vi "motor.vi"() -> ()   [LabVIEW 2016]
uses:
  <vilib>/myRIO/Common/Instrument Driver Framework/myRIO v1.0/Encoder/typedefs/Encoder Signal Mode.ctl
  <vilib>/myRIO/Instrument Drivers/Onboard IO/DIO/typedefs/DIO Reference.ctl
  <vilib>/myRIO/Common/Instrument Driver Framework/Utilities/typedefs/myRIO Generic Hardware Reference.ctl
  <vilib>/myRIO/Common/Instrument Driver Framework/Utilities/typedefs/Hardware Version Enum.ctl
  <vilib>/myRIO/Common/Instrument Driver Framework/Utilities/typedefs/myRIO v1.0 Reference.ctl
  <vilib>/myRIO/Common/Instrument Driver Framework/Utilities/typedefs/Generic FPGA Reference.ctl
  <vilib>/myRIO/Common/Instrument Driver Framework/myRIO v1.0/DIO/typedefs/DIO Channels List.ctl
  <vilib>/myRIO/Common/Instrument Driver Framework/myRIO v1.0/DIO/typedefs/DIO Channels Enum.ctl
  <vilib>/userdefined/High Color/nirio_resource_hc.ctl
  <vilib>/myRIO/Instrument Drivers/Onboard IO/PWM/typedefs/PWM Reference.ctl
  <vilib>/myRIO/Common/Instrument Driver Framework/myRIO v1.0/PWM/typedefs/PWM Channels Enum.ctl
  <vilib>/myRIO/Instrument Drivers/Onboard IO/PWM/typedefs/PWM Configuration.ctl
  <vilib>/myRIO/Common/Instrument Driver Framework/myRIO v1.0/Encoder/typedefs/Encoder Configuration v1.0.ctl
  <vilib>/myRIO/Instrument Drivers/Onboard IO/Encoder/typedefs/Encoder Reference.ctl
  <vilib>/myRIO/Common/Instrument Driver Framework/myRIO v1.0/Encoder/typedefs/Encoder Channels Enum.ctl
  <vilib>/myRIO/Common/Instrument Driver Framework/Utilities/vis/Is FPGA Ref Available.vi
  <vilib>/myRIO/Common/Instrument Driver Framework/myRIO v1.0/DIO/vis/myRIO v1.1 Open DIO.vi
  <vilib>/myRIO/Instrument Drivers/Onboard IO/DIO/vis/Write.vi
  <vilib>/myRIO/Common/Instrument Driver Framework/myRIO v1.0/PWM/vis/myRIO v1.1 Open PWM.vi
  <vilib>/myRIO/Common/Instrument Driver Framework/myRIO v1.0/Encoder/vis/myRIO v1.1 Open Encoder.vi
  <vilib>/myRIO/Common/Instrument Driver Framework/Utilities/vis/Validate Channels.vi
  <vilib>/myRIO/Common/Instrument Driver Framework/myRIO v1.0/DIO/vis/myRIO v1.0 Reserve DIO.vi
  <vilib>/myRIO/Common/Instrument Driver Framework/myRIO v1.0/PWM/vis/myRIO v1.0 Reserve PWM.vi
  <vilib>/myRIO/Common/Instrument Driver Framework/myRIO v1.0/Encoder/vis/myRIO v1.0 Reserve Encoder.vi
  <vilib>/myRIO/Common/Instrument Driver Framework/myRIO v1.0/Encoder/vis/myRIO v1.0 Close Encoder.vi
  <vilib>/myRIO/Common/Instrument Driver Framework/myRIO v1.0/PWM/vis/myRIO v1.0 Close PWM.vi
  <vilib>/myRIO/Common/Instrument Driver Framework/myRIO v1.0/Resource Manager/vis/myRIO v1.0 Reserve Channel List.vi
  <vilib>/myRIO/Common/Instrument Driver Framework/myRIO v1.0/DIO/vis/myRIO v1.0 Build MUX Configuration DIO.vi
  <vilib>/myRIO/Common/Instrument Driver Framework/myRIO v1.0/PWM/vis/myRIO v1.0 Build MUX Configuration PWM.vi
  <vilib>/myRIO/Common/Instrument Driver Framework/myRIO v1.0/Encoder/vis/myRIO v1.0 Build MUX Configuration Encoder.vi
  <vilib>/myRIO/Common/Instrument Driver Framework/myRIO v1.0/Encoder/vis/myRIO v1.0 Unreserve Encoder.vi
  <vilib>/myRIO/Common/Instrument Driver Framework/myRIO v1.0/PWM/vis/myRIO v1.0 Unreserve PWM.vi
  <vilib>/myRIO/Common/Instrument Driver Framework/myRIO v1.0/Resource Manager/vis/myRIO v1.0 Reserve Channel.vi
  <vilib>/myRIO/Common/Instrument Driver Framework/myRIO v1.0/Resource Manager/vis/myRIO v1.0 Unreserve Channel.vi
  <vilib>/myRIO/Common/Instrument Driver Framework/myRIO v1.0/Resource Manager/vis/myRIO v1.0 Create Configuration List.vi
  <vilib>/myRIO/Common/Instrument Driver Framework/myRIO v1.0/Resource Manager/vis/myRIO v1.0 Unreserve Channel List.vi
  <vilib>/myRIO/Common/Instrument Driver Framework/myRIO v1.0/Resource Manager/vis/myRIO v1.0 Build Mutex Name.vi
  <vilib>/Utility/VariantDataType/GetNumericInfo.vi
  <vilib>/Utility/error.llb/Error Cluster From Error Code.vi
  <vilib>/myRIO/Common/Instrument Driver Framework/myRIO v1.0/myRIO v1.1 Open.vi
  <vilib>/myRIO/Common/Instrument Driver Framework/Utilities/vis/IO Manager.vi
  <vilib>/myRIO/Common/Instrument Driver Framework/Utilities/vis/Configuration Manager.vi
  <vilib>/myRIO/Common/Instrument Driver Framework/myRIO v1.0/Resource Manager/vis/myRIO v1.0 Configure IO.vi
  <vilib>/myRIO/Common/Instrument Driver Framework/myRIO v1.0/myRIO v1.0 Close.vi
  <vilib>/myRIO/Common/Instrument Driver Framework/myRIO v1.0/DIO/vis/myRIO v1.0 Write DIO.vi
  <vilib>/myRIO/Common/Instrument Driver Framework/myRIO v1.0/Encoder/vis/myRIO v1.0 Configure Encoder.vi
  <vilib>/myRIO/Common/Instrument Driver Framework/myRIO v1.0/Encoder/vis/myRIO v1.0 Read Encoder.vi
  <vilib>/addons/control/pid/pid.llb/PID (DBL).vi
  <vilib>/myRIO/Common/Instrument Driver Framework/myRIO v1.0/PWM/vis/myRIO v1.0 Write PWM.vi
  <vilib>/myRIO/Common/Instrument Driver Framework/myRIO v1.0/Encoder/vis/myRIO v1.0 Shutdown Encoder.vi
  <vilib>/myRIO/Common/Instrument Driver Framework/myRIO v1.0/PWM/vis/myRIO v1.0 Shutdown PWM.vi
  <vilib>/myRIO/Express VI/Onboard IO/DO/DO Express VI.xnode
  <vilib>/myRIO/Instrument Drivers/Onboard IO/DIO/vis/myRIO DIO Open.xnode
  <vilib>/myRIO/Instrument Drivers/Onboard IO/Encoder/vis/myRIO Encoder Open.xnode
  <vilib>/myRIO/Instrument Drivers/Onboard IO/PWM/vis/myRIO PWM Open.xnode
  <vilib>/myRIO/Instrument Drivers/Onboard IO/Encoder/Encoder.lvlib
  <vilib>/myRIO/Instrument Drivers/Onboard IO/PWM/PWM.lvlib
  <vilib>/myRIO/Instrument Drivers/Onboard IO/DIO/DIO.lvlib
  <vilib>/addons/control/pid/NI_PID_pid.lvlib
panel:
  out "element":dbl
  in  "Numeric":dbl
  in  "PID gains":T1={"proportional gain (Kc)"=1.0, "integral time (Ti, min)"=0.01, "derivative time (Td, min)"=0.0} {"derivative time (Td, min)" format="%.6f"; "integral time (Ti, min)" format="%.6f"; "proportional gain (Kc)" format="%.4f"}
  out "Waveform Chart":dbl(graph)
  in  "Boolean 2":bool
  out "error out 4":errorcluster
  in  "error in (no error) 4":errorcluster
  in  "Boolean":bool
  out "error out 3":errorcluster
  in  "error in (no error) 3":errorcluster
  out "error out 2":errorcluster
  in  "error in (no error)":errorcluster
  out "Counter Value":i32
  in  "stop":bool
  out "error out":errorcluster
  in  "error in (no error) 2":errorcluster
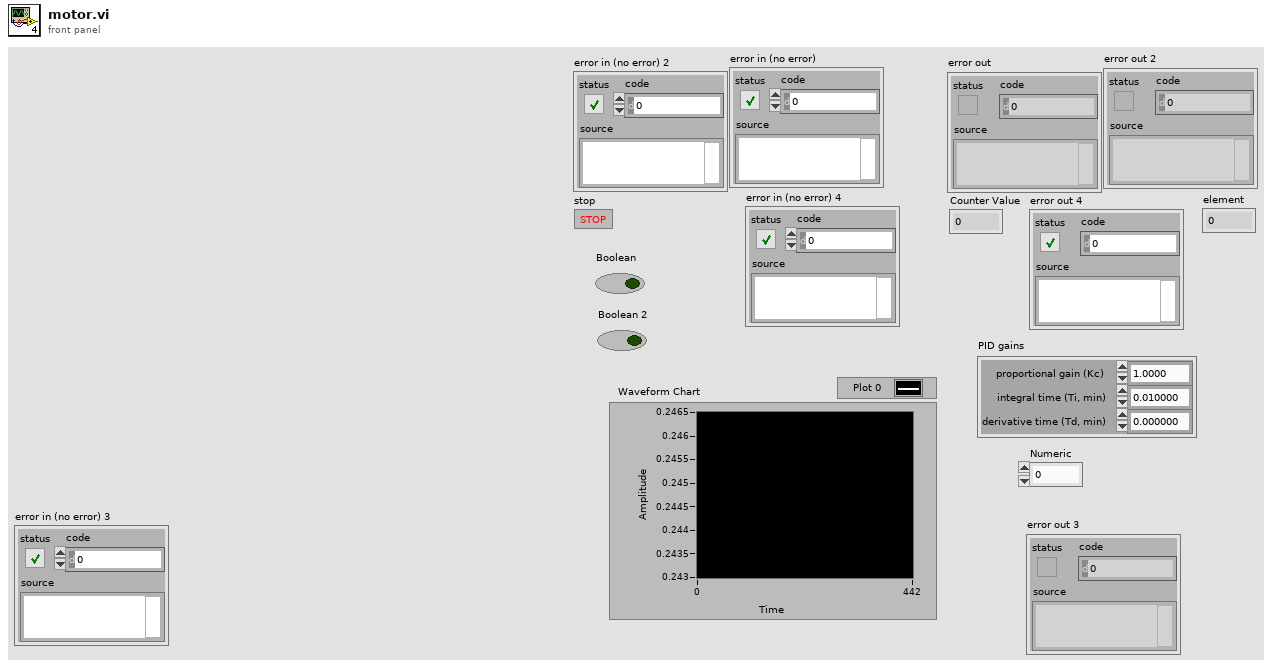
[diagram p1: front panel]
types:
  T1 = cluster{"proportional gain (Kc)":dbl, "integral time (Ti, min)":dbl, "derivative time (Td, min)":dbl}
  T2 = typedef "Encoder Signal Mode.ctl" = enum16{"Quadrature phase signal", "Step and direction signal"}
  T3 = typedef "DIO.lvlib/DIO Reference.ctl" = cluster{"myRIO Reference":T4, "DIO Channels List":T8}
  T4 = typedef "myRIO Generic Hardware Reference.ctl" = cluster{"myRIO Model":T5, "myRIO Hardware Reference":T6}
  T5 = typedef "Hardware Version Enum.ctl" = enum16{"Unknown", "myRIO-1900", "myRIO-1950", "roboRIO", "NI ELVIS RIO CM"}
  T6 = typedef "myRIO v1.0 Reference.ctl" = cluster{"Generic FPGA Reference":T7, "Allow multiple opens":bool}
  T7 = typedef "Generic FPGA Reference.ctl" = refnum<k20>
  T8 = typedef "DIO Channels List.ctl" = T9[]
  T9 = typedef "DIO Channels Enum.ctl" = enum16{"Not Connected", "C/DIO0", "C/DIO1", "C/DIO2", "C/DIO3", "C/DIO4", "C/DIO5", "C/DIO6", "C/DIO7", "A/DIO0", "A/DIO1", "A/DIO2", "A/DIO3", "A/DIO4", "A/DIO5", "A/DIO6", "A/DIO7", "A/DIO8", "A/DIO9", "A/DIO10", "A/DIO11", "A/DIO12", "A/DIO13", "A/DIO14", "A/DIO15", "B/DIO0", "B/DIO1", "B/DIO2", "B/DIO3", "B/DIO4", "B/DIO5", "B/DIO6", "B/DIO7", "B/DIO8", "B/DIO9", "B/DIO10", "B/DIO11", "B/DIO12", "B/DIO13", "B/DIO14", "B/DIO15", "LED0", "LED1", "LED2", "LED3", "Button0", "DIO/DIO0", "DIO/DIO1", "DIO/DIO2", "DIO/DIO3", "DIO/DIO4", "DIO/DIO5", "DIO/DIO6", "DIO/DIO7", "DIO/DIO8", "DIO/DIO9", "SPI/CS0", "SPI/CS1", "SPI/CS2", "SPI/CS3", "LED RADIO (Green)", "LED RADIO (Red)", "LED COMM (Green)", "LED COMM (Red)", "LED MODE (Green)", "LED MODE (Red)"}
  T10 = typedef "nirio_resource_hc.ctl" = tag
  T11 = typedef "PWM.lvlib/PWM Reference.ctl" = cluster{"myRIO Reference":T4, "PWM Channels Enum":T12, "PWM Configuration":T13}
  T12 = typedef "PWM Channels Enum.ctl" = enum16{"Not Connected", "C/PWM0", "C/PWM1", "A/PWM0", "A/PWM1", "A/PWM2", "B/PWM0", "B/PWM1", "B/PWM2", "PWM/PWM0", "PWM/PWM1", "PWM/PWM2", "PWM/PWM3", "PWM/PWM4", "PWM/PWM5", "PWM/PWM6", "PWM/PWM7", "PWM/PWM8", "PWM/PWM9"}
  T13 = typedef "PWM.lvlib/PWM Configuration.ctl" = cluster{"Frequency":dbl, "Duty Cycle":dbl}
  T14 = typedef "Encoder.lvlib/Encoder Reference.ctl" = cluster{"myRIO Reference":T4, "Encoder Channels Enum":T15}
  T15 = typedef "Encoder Channels Enum.ctl" = enum16{"Not Connected", "C/ENC0", "C/ENC1", "A/ENC", "B/ENC", "DIO/ENC0", "DIO/ENC1", "DIO/ENC2", "DIO/ENC3", "DIO/ENC4"}
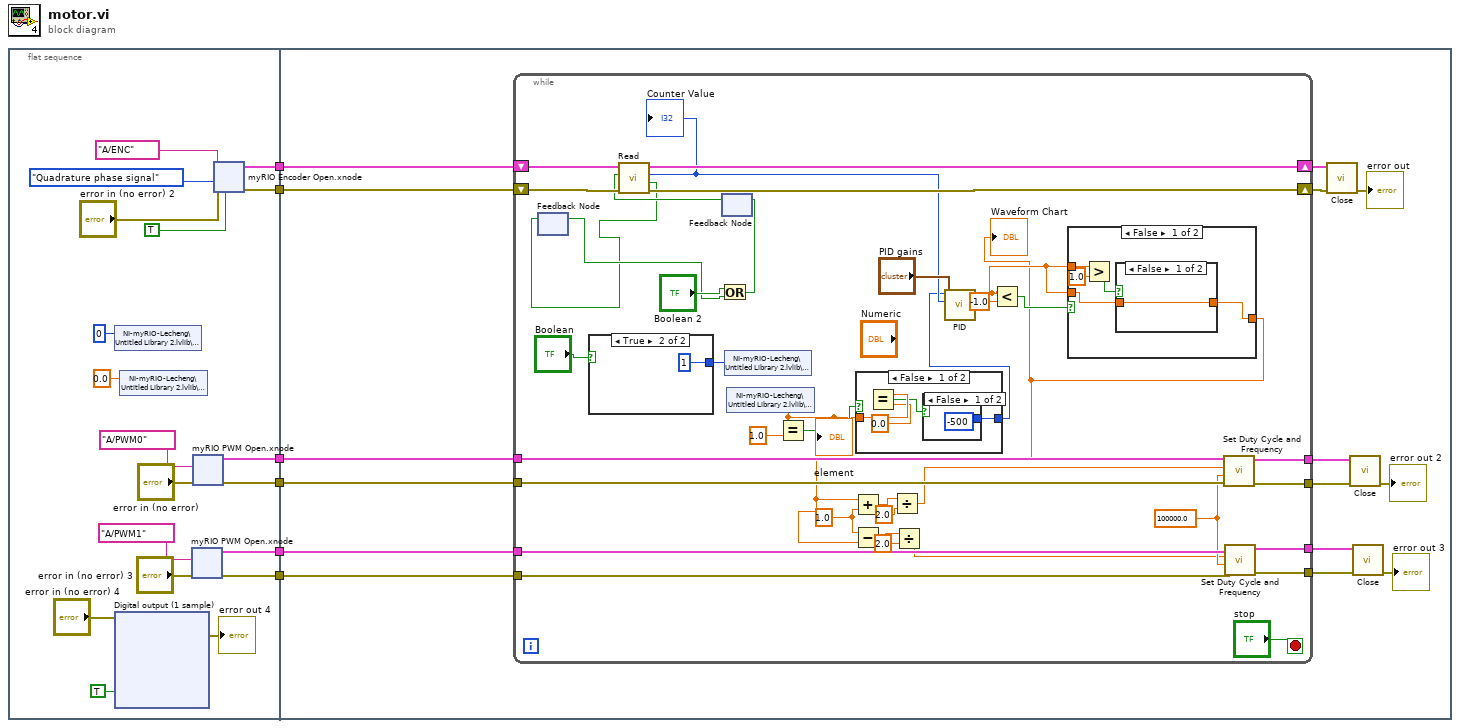
[diagram p0: block diagram]
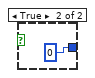
[diagram p2: hidden frame]
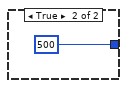
[diagram p3: hidden frame]
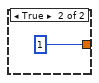
[diagram p4: hidden frame]
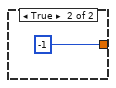
[diagram p5: hidden frame]
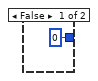
[diagram p6: hidden frame]
diagram:
  n1 = flat-sequence {
    tunnel: [w17] -> w6
    tunnel: [w16] -> w5
    tunnel: [w15] -> w4
    tunnel: [w14] -> w3
    tunnel: [w13] -> w2
    tunnel: [w12] -> w1
    tunnel: w6 -> [w119]
    tunnel: w5 -> [w118]
    tunnel: w4 -> [w117]
    tunnel: w3 -> [w116]
    tunnel: w2 -> [w115]
    tunnel: w1 -> [w114]
    frame #0 {
      n2 = shared-variable "NI-myRIO-Lecheng\\Untitled Library 2.lvlib\\Variable"(0 ("Variable")) -> ()  [unwired: 1 in, 1 out]
      n3 = xnode "Digital output (1 sample)"("B/DIO0 (Pin 11)"=TRUE, "error in (no error)"="error in (no error) 4") -> ("error out"=→"error out 4":errorcluster)
      n4 = shared-variable "NI-myRIO-Lecheng\\Untitled Library 2.lvlib\\element"(0.0 ("element")) -> ()  [unwired: 1 in, 1 out]
      n5 = xnode "myRIO PWM Open.xnode"("error in (no error)"="error in (no error) 3", "Channel Name"=tag "A/PWM1") -> ("error out"=w16:errorcluster, "PWM Ref Out"=w17:T11)  [unwired: 1 in]
      n6 = xnode "myRIO PWM Open.xnode"("error in (no error)"="error in (no error)", "Channel Name"=tag "A/PWM0") -> ("error out"=w15:errorcluster, "PWM Ref Out"=w14:T11)  [unwired: 1 in]
      n7 = xnode "myRIO Encoder Open.xnode"("error in (no error)"="error in (no error) 2", "Channel Name"=tag "A/ENC", "Start Counter"=TRUE, "Encoder Signal Mode"=Encoder_Signal_Mode."Quadrature phase signal") -> ("error out"=w13:errorcluster, "Encoder Ref Out"=w12:T14)  [unwired: 1 in]
    }
    frame #1 {
      n8 = while {
        shift-right: [w163] -> w127
        shift-left: w114 -> [w166]
        shift-right: [w164] -> w128
        shift-left: w115 -> [w165]
        tunnel: w116 -> [w161]
        tunnel: w117 -> [w160]
        tunnel: [w159] -> w125
        tunnel: [w158] -> w124
        tunnel: w118 -> [w157]
        tunnel: w119 -> [w156]
        tunnel: [w155] -> w121
        tunnel: [w154] -> w120
        stop <- "stop" stop-if-true
        w152 = 1.0 ("y")
        w153 = 100000.0 ("Frequency [Hz]")
        n9 = feedback #1() -> (w138:bool)  [unwired: 1 in]
        n10 = case shown="True" "Boolean" {
          tunnel: [0 1] -> w144
          frame False {
          }
          frame True {
          }
        }
        n11 = Or(x="Boolean 2", y=w138) -> (x .or. y?=w134:bool)
        n12 = feedback-in #2(w134) -> ()
        n13 = feedback #2() -> (w136:bool)  [unwired: 1 in]
        n14 = call <vilib>:"Read.vi"("error in (no error)"=w165, "Reset Counter"=w136, "Encoder Ref In"=w166) -> ("error out"=w164:errorcluster, "Overflow?"=w133:bool, "Counter Value"=w137:i32, "Encoder Ref Out"=w163:T14)  [unwired: 4 in, 1 out]
        "Counter Value" <- w137
        n15 = feedback-in #1(w133) -> ()
        n16 = shared-variable "NI-myRIO-Lecheng\\Untitled Library 2.lvlib\\Variable"(w144) -> ()  [unwired: 1 in, 1 out]
        n17 = shared-variable "NI-myRIO-Lecheng\\Untitled Library 2.lvlib\\element"() -> (w129:dbl)  [unwired: 1 in, 1 out]
        "element" <- w129
        n18 = Equal?(x=w129, y=1.0) -> (x = y?=w131:bool)
        n19 = case shown="False" w131 {
          tunnel: [w167 500] -> w130
          tunnel: w129 -> [w170 _]
          frame False {
            n20 = Equal?(x=w170, y=0.0) -> (x = y?=w168:bool)
            n21 = case shown="False" w168 {
              tunnel: [-500 0] -> w167
              frame False {
              }
              frame True {
              }
            }
          }
          frame True {
          }
        }
        n22 = call-poly <vilib>:"PID.vi"("PID gains"="PID gains", "process variable"=w137, "setpoint"=w130) -> ("output"=w141:dbl)  [unwired: 7 in, 1 out]
        n23 = Less?(x=w141, y=-1.0) -> (x < y?=w142:bool)
        n24 = case shown="False" w142 {
          tunnel: [w175 -1] -> w135
          tunnel: w141 -> [w178 _]
          tunnel: w141 -> [w174 _]
          frame False {
            n25 = Greater?(x=w178, y=1.0) -> (0:w176:bool)
            n26 = case shown="False" w176 {
              tunnel: [w179 1] -> w175
              tunnel: w174 -> [w179 _]
              frame False {
              }
              frame True {
              }
            }
          }
          frame True {
          }
        }
        "Waveform Chart" <- w135
        n27 = Add(x=w135, y=w152) -> (x+y=w151:dbl)
        n28 = Subtract(x=w152, y=w135) -> (x-y=w149:dbl)
        n29 = Divide(x=w151, y=2.0) -> (x/y=w147:dbl)
        n30 = Divide(x=w149, y=2.0) -> (x/y=w146:dbl)
        n31 = call <vilib>:"Set Duty Cycle and Frequency.vi"("error in (no error)"=w160, "Frequency [Hz]"=w153, "Duty Cycle"=w147, "PWM Ref In"=w161) -> ("error out"=w159:errorcluster, "PWM Ref Out"=w158:T11)  [unwired: 5 in]
        n32 = call <vilib>:"Set Duty Cycle and Frequency.vi"("error in (no error)"=w157, "Frequency [Hz]"=w153, "Duty Cycle"=w146, "PWM Ref In"=w156) -> ("error out"=w154:errorcluster, "PWM Ref Out"=w155:T11)  [unwired: 5 in]
      }
      n33 = call <vilib>:"Close.vi"("error in (no error)"=w128, "Encoder Ref In"=w127) -> ("error out"=→"error out":errorcluster)  [unwired: 9 in]
      n34 = call <vilib>:"Close.vi"("error in (no error)"=w125, "PWM Ref In"=w124) -> ("error out"=→"error out 2":errorcluster)  [unwired: 9 in]
      n35 = call <vilib>:"Close.vi"("error in (no error)"=w120, "PWM Ref In"=w121) -> ("error out"=→"error out 3":errorcluster)  [unwired: 9 in]
    }
  }
